vi "Get Error.vi"(8 "error in (no error)":errorcluster) -> (0 "error out":errorcluster, 3 "lpBuffer":string)   [LabVIEW 2013]
uses:
  kernel32.dll
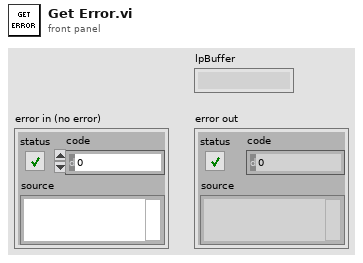
[diagram p1: front panel]
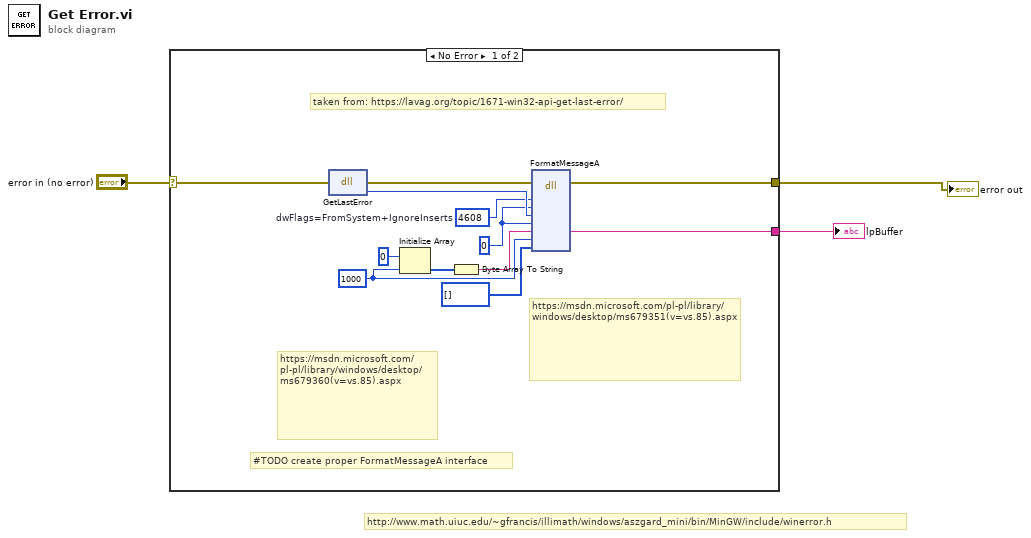
[diagram p0: block diagram]
diagram:
  # "http://www.math.uiuc.edu/~gfrancis/illimath/windows/aszgard_mini/bin/MinGW/include/winerror.h"
  n1 = case shown="No Error" "error in (no error)" {
    selector: "error in (no error)" -> [w4 w16]
    tunnel: [w7 _] -> w3
    tunnel: [w5 w16] -> w2
    frame No Error {
      w9 = u32 1000 ("Dimension Size")
      w6 = u32 0 ("lpSource")
      w13 = u32 4608  # dwFlags=FromSystem+IgnoreInserts
      # "#TODO create proper FormatMessageA interface"
      # "taken from: https://lavag.org/topic/1671-win32-api-get-last-error/"
      # "https://msdn.microsoft.com/pl-pl/library/windows/desktop/ms679360(v=vs.85).aspx"
      # "https://msdn.microsoft.com/pl-pl/library/windows/desktop/ms679351(v=vs.85).aspx"
      n2 = dll-call lib="kernel32.dll" fn="GetLastError"(error in=w4) -> (error out=w15:errorcluster, "return type"=w14:u32)  [unwired: 2 in, 1 out]
      n3 = Initialize Array(u8 0 ("Element Data"), w9) -> (w10:u8[])
      n4 = Byte Array To String(unsigned byte array=w10) -> (string=w11:string)
      n5 = dll-call lib="kernel32.dll" fn="FormatMessageA"(error in=w15, "dwFlags"=w13, "lpSource"=w6, "dwMessageId"=w14, "dwLanguageId"=w6, "lpBuffer"=w11, "nSize"=w9, "Arguments"=u8[] []) -> (error out=w5:errorcluster, "lpBuffer"=w7:string)  [unwired: 9 in, 1 out]
    }
    frame Error {
    }
  }
  "lpBuffer" <- w3
  "error out" <- w2
